vi "MSGR Object Registry.vi"(7 "function (get data)":T3=enum."get data", 8 "error in (no error)":errorcluster, 10 "MSGR Q":T1, 11 "MSGR Q name":T2) -> (0 "error out":errorcluster, 1 "MSGR Q names":T2[](array[typedef]), 2 "MSGR Q":T1, 3 "MSGR Q name":T2, 4 "valid index?":bool)   [LabVIEW 2018]
doc: "$Author::Richard Jennings $\n$Rev:: $\n$Date:: May, 2008 $\n\nOVERVIEW:\nReentrant VI to receive messages via a MSGR Q. If the Q does not exist this VI will create it, then wait for data.\n\nINPUTS (Controls):\n<name> - <short description of each control wired to connector pane>\n\nOUTPUTS (Indicators):\n<name> - <short description of each indicator wired to connector pane>\n\nCopyright 2008 - 2017 Jennings Embedded Servies. All rights reserved.\nAuthor makes no warranties or guarantees related to performance of the software.\nUSE AT YOUR OWN RISK\nwww.jembedded.com"
uses:
  MSGR Q Name TypeDef.ctl
  MSGR Registry Control TypeDef.ctl
  MSGR Q Ref TypeDef.ctl
  MSGR Q Data TypeDef.ctl
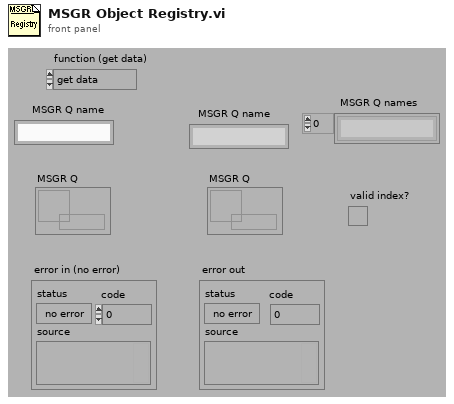
[diagram p1: front panel]
types:
  T1 = typedef "MSGR Q Ref TypeDef.ctl" = refnum<queue>
  T2 = typedef "MSGR Q Name TypeDef.ctl" = string
  T3 = typedef "MSGR Registry Control TypeDef.ctl" = enum16{"reset", "register", "get data", "set data", "unregister", "test", "get objects"}
  T4 = enum16{"reset", "register", "get data", "set data", "unregister", "test", "get objects"}
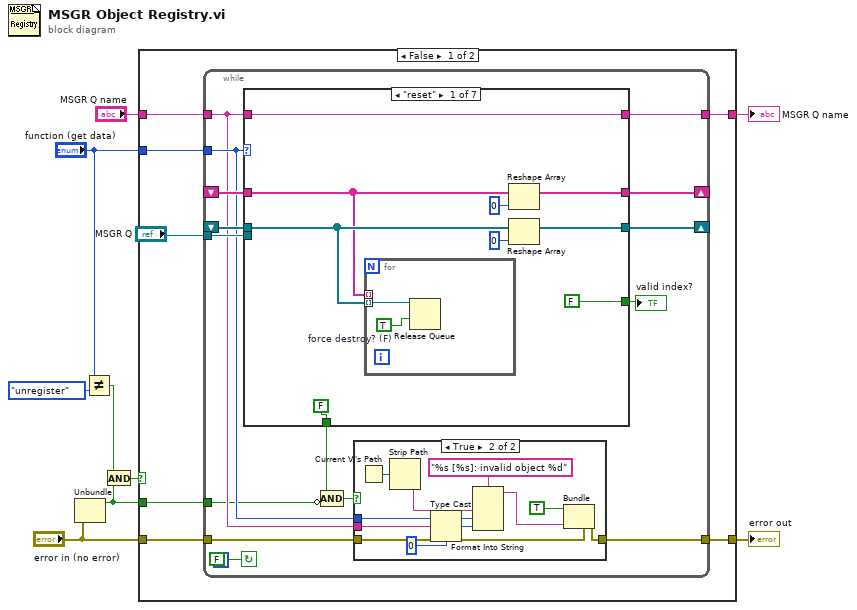
[diagram p0: block diagram]
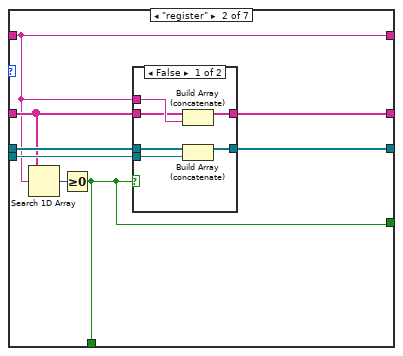
[diagram p3: hidden frame]
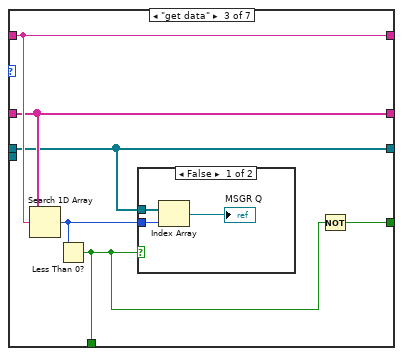
[diagram p5: hidden frame]
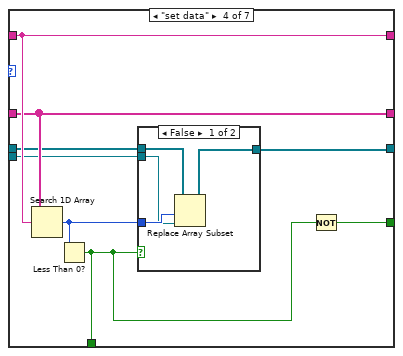
[diagram p7: hidden frame]
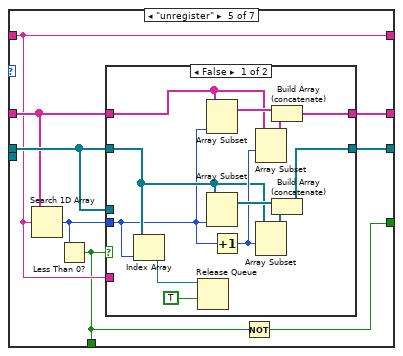
[diagram p9: hidden frame]
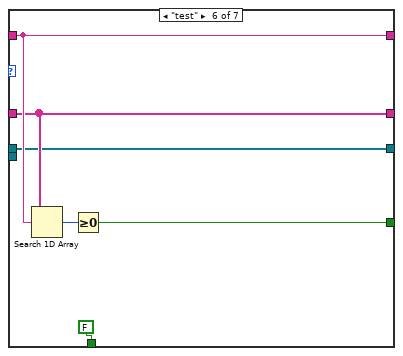
[diagram p11: hidden frame]
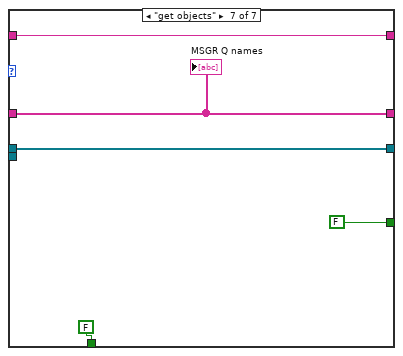
[diagram p12: hidden frame]
diagram:
  n1 = Unbundle("error in (no error)") -> ("status"=w1:bool)  [unwired: 2 out]
  n2 = Not Equal?(x="function (get data)", y=T4."unregister" ("function (get data)")) -> (x != y?=w2:bool)
  n3 = And(x=w2, y=w1) -> (x .and. y?=w3:bool)
  n4 = case shown="False" w3 {
    tunnel: "error in (no error)" -> [w16 w127]
    tunnel: [w15 w126] -> w9
    tunnel: [w14 w127] -> w7
    tunnel: "MSGR Q name" -> [w13 w126]
    tunnel: "function (get data)" -> [w12 _]
    tunnel: w1 -> [w11 _]
    frame False {
      n5 = while {
        tunnel: w11 -> [w20]
        tunnel: [w22] -> w14
        tunnel: w16 -> [w23]
        tunnel: "MSGR Q" -> [w26]
        tunnel: w12 -> [w25]
        tunnel: [w27] -> w15
        tunnel: w13 -> [w24]
        shift-left: _ -> [w29]
        shift-right: [w28] -> _
        shift-left: _ -> [w31]
        shift-right: [w30] -> _
        stop <- FALSE continue-if-true
        n6 = case shown="\"reset\"" w25 {
          tunnel: w31 -> [w45 w57 w75 w86 w98 w118 w125]
          tunnel: w24 -> [w48 w56 w76 w87 w95 w120 w123]
          tunnel: [w48 w56 w76 w87 w95 w120 w123] -> w27
          tunnel: [w49 w62 w75 w86 w97 w118 w125] -> w30
          tunnel: [w52 w60 w73 w83 w96 w117 w124] -> w28
          tunnel: w29 -> [w46 w61 w73 w84 w99 w117 w124]
          tunnel: w26 -> [_ w59 _ w82 _ _ _]
          tunnel: [FALSE w55 w72 w81 w94 FALSE FALSE] -> w21
          tunnel: [FALSE w55 w71 w80 w93 w115 FALSE] -> w17
          frame "reset" {
            n7 = for {
              tunnel: w46 -> [w54] mode=indexing
              tunnel: w45 -> [_] mode=indexing
              w53 = TRUE  # force destroy? (F)
              n8 = Release Queue(queue=w54, force destroy? (F)=w53) -> ()  [unwired: 1 in, 3 out]
            }
            n9 = Reshape Array(w45, 0) -> (w49:T2[])
            n10 = Reshape Array(w46, 0) -> (w52:T1[])
          }
          frame "register" {
            n11 = Search 1D Array(1D array=w57, element=w56) -> (index of element=w58:i32)  [unwired: 1 out]
            n12 = Greater Or Equal To 0?(x=w58) -> (x >= 0?=w55:bool)
            n13 = case shown="False" w55 {
              tunnel: w56 -> [w68 _]
              tunnel: w57 -> [w67 w70]
              tunnel: w59 -> [w66 _]
              tunnel: [w65 w69] -> w60
              tunnel: w61 -> [w64 w69]
              tunnel: [w63 w70] -> w62
              frame False {
                n14 = Build Array (concatenate)(w67, w68) -> (w63:T2[])
                n15 = Build Array (concatenate)(w64, w66) -> (w65:T1[])
              }
              frame True {
              }
            }
          }
          frame "get data" {
            n16 = Search 1D Array(1D array=w75, element=w76) -> (index of element=w74:i32)  [unwired: 1 out]
            n17 = Less Than 0?(x=w74) -> (x < 0?=w72:bool)
            n18 = case shown="False" w72 {
              tunnel: w74 -> [w79 _]
              tunnel: w73 -> [w78 _]
              frame False {
                n19 = Index Array(array=w78, index=w79) -> (element=→"MSGR Q":T1)
              }
              frame True {
              }
            }
            n20 = Not(x=w72) -> (.not. x?=w71:bool)
          }
          frame "set data" {
            n21 = Search 1D Array(1D array=w86, element=w87) -> (index of element=w85:i32)  [unwired: 1 out]
            n22 = Less Than 0?(x=w85) -> (x < 0?=w81:bool)
            n23 = case shown="False" w81 {
              tunnel: w85 -> [w91 _]
              tunnel: w84 -> [w90 w92]
              tunnel: w82 -> [w89 _]
              tunnel: [w88 w92] -> w83
              frame False {
                n24 = Replace Array Subset(array=w90, new element=w89, index=w91) -> (w88:T1[])
              }
              frame True {
              }
            }
            n25 = Not(x=w81) -> (.not. x?=w80:bool)
          }
          frame "unregister" {
            n26 = Search 1D Array(1D array=w98, element=w95) -> (index of element=w100:i32)  [unwired: 1 out]
            n27 = Less Than 0?(x=w100) -> (x < 0?=w94:bool)
            n28 = case shown="False" w94 {
              tunnel: w100 -> [w103 _]
              tunnel: w99 -> [_ _]
              tunnel: w99 -> [w104 w113]
              tunnel: w98 -> [w107 w114]
              tunnel: [w106 w114] -> w97
              tunnel: [w105 w113] -> w96
              tunnel: w95 -> [_ _]
              frame False {
                n29 = Index Array(array=w104, index=w103) -> (element=w102:T1)
                n30 = Release Queue(queue=w102, force destroy? (F)=TRUE) -> ()  [unwired: 1 in, 3 out]
                n31 = Array Subset(array=w107, length=w103) -> (w109:T2[])  [unwired: 1 in]
                n32 = Array Subset(array=w104, length=w103) -> (w112:T1[])  [unwired: 1 in]
                n33 = Increment(x=w103) -> (x+1=w108:i32)
                n34 = Array Subset(array=w107, index=w108) -> (w110:T2[])  [unwired: 1 in]
                n35 = Array Subset(array=w104, index=w108) -> (w111:T1[])  [unwired: 1 in]
                n36 = Build Array (concatenate)(w109, w110) -> (w106:T2[])
                n37 = Build Array (concatenate)(w112, w111) -> (w105:T1[])
              }
              frame True {
              }
            }
            n38 = Not(x=w94) -> (.not. x?=w93:bool)
          }
          frame "test" {
            n39 = Search 1D Array(1D array=w118, element=w120) -> (index of element=w119:i32)  [unwired: 1 out]
            n40 = Greater Or Equal To 0?(x=w119) -> (x >= 0?=w115:bool)
          }
          frame "get objects" {
            "MSGR Q names" <- w125
          }
        }
        "valid index?" <- w17
        n41 = Compound Arithmetic op=AND(w21, invert w20) -> (w19:bool)
        n42 = case shown="True" w19 {
          tunnel: w25 -> [_ w41]
          tunnel: w24 -> [_ w42]
          tunnel: w23 -> [w32 w40]
          tunnel: [w32 w37] -> w22
          frame False {
          }
          frame True {
            n43 = Current VI's Path() -> (path=w36:path)
            n44 = Strip Path(path=w36) -> (name=w35:string)  [unwired: 1 out]
            n45 = Type Cast(type=u32 0 ("object"), x=w42) -> (*(type *) &x=w34:u32)
            n46 = Format Into String(format string="%s [%s]: invalid object %d", w35, w41, w34) -> (resulting string=w39:string)  [unwired: 2 in, 1 out]
            n47 = Bundle(cluster=w40, "status"=TRUE, "source"=w39) -> (w37:errorcluster)  [unwired: 1 out]
          }
        }
      }
    }
    frame True {
    }
  }
  "MSGR Q name" <- w9
  "error out" <- w7
